vi "_Raise WebMessageReceived.vi"(4 "Display State In":T1, 5 "Event Data":cluster{"sender":refnum<k24>, "e":refnum<k24>}, 6 "Control Ref":refnum<k24>, 7 "Event Common Data":T2) -> ()   [LabVIEW 2020, in "WebView2 Control.xctl"]
uses:
  WebView2 Control.xctl
  C:/Users/kleins/Desktop/webview2/microsoft.web.webview2.1.0.1370.28/lib/net45/Microsoft.Web.WebView2.Core.dll
  microsoft.web.webview2.1.0.1370.28/lib/net45/Microsoft.Web.WebView2.Core.dll
  Events.ctl
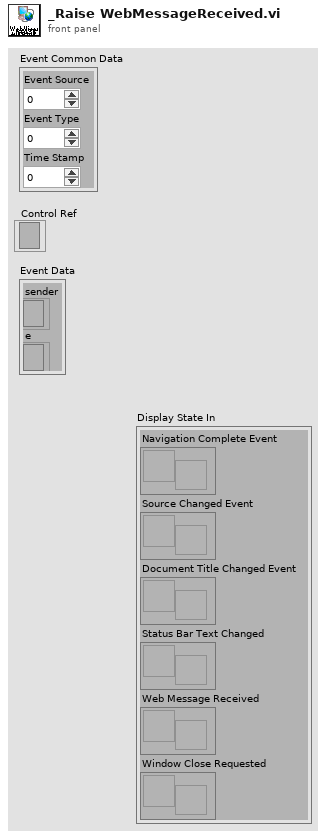
[diagram p1: front panel]
types:
  T1 = typedef "WebView2 Control.xctl/Events.ctl" = cluster{"Navigation Complete Event":refnum<user-event>, "Source Changed Event":refnum<user-event>, "Document Title Changed Event":refnum<user-event>, "Status Bar Text Changed":refnum<user-event>, "Web Message Received":refnum<user-event>, "Window Close Requested":refnum<user-event>}
  T2 = cluster{"Event Source":i32, "Event Type":u32, "Time Stamp":u32}
  T3 = cluster{"Source":string, "WebMessageAsJson":string}
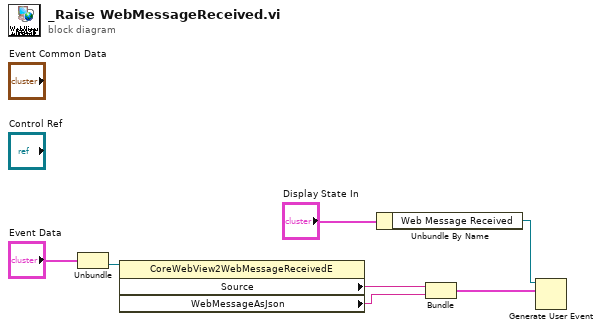
[diagram p0: block diagram]
diagram:
  n1 = Unbundle("Event Data") -> ("e"=w4:refnum<k24>)  [unwired: 1 out]
  n2 = property class="CoreWebView2WebMessageReceivedE"(reference=w4) -> ("Source"=w3:string, "WebMessageAsJson"=w2:string)  [unwired: 1 in, 2 out]
  n3 = Unbundle By Name("Display State In") -> ("Web Message Received"=w5:refnum<user-event>)
  n4 = Bundle("Source"=w3, "WebMessageAsJson"=w2) -> (w1:T3)  [unwired: 1 in]
  n5 = Generate User Event(user event=w5, event data cluster=w1) -> ()  [unwired: 2 in, 2 out]
